vi "CRYGet Weight Array Value.vi"(8 "spectrum type":enum16{"Power", "Amplitude"}(ring), 9 "dB On (T)":bool=TRUE, 10 "frequency [Hz]":dbl=1000.0 min=0.0 format="%.2f", 11 "weighting enum":T1(ring)) -> (3 "relative response level":dbl format="%.2f")   [LabVIEW 2013]
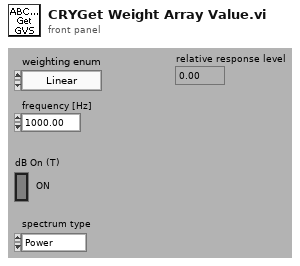
[diagram p1: front panel]
types:
  T1 = enum16{"Linear", "A-weighting", "B-weighting", "C-weighting", "ITU-R 468-4", "Dolby", "CCITT", "C-message", "Wb", "Wc", "Wd", "We", "Wf", "Wh", "Wj", "Wk", "Wm", "Undefined"}
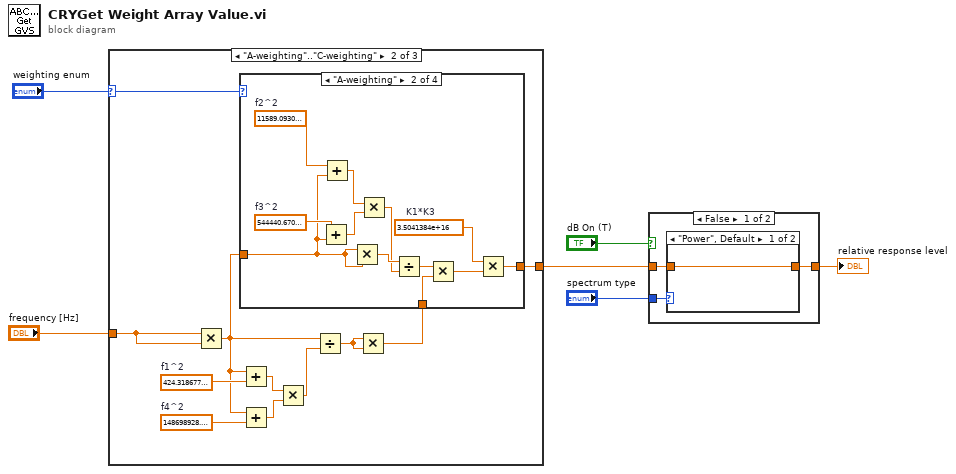
[diagram p0: block diagram]
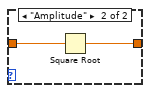
[diagram p2: hidden frame]
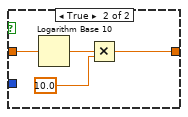
[diagram p3: hidden frame]
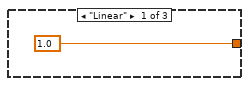
[diagram p4: hidden frame]
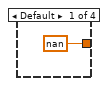
[diagram p5: hidden frame]
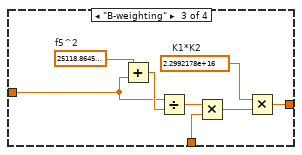
[diagram p6: hidden frame]
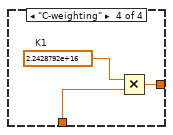
[diagram p7: hidden frame]
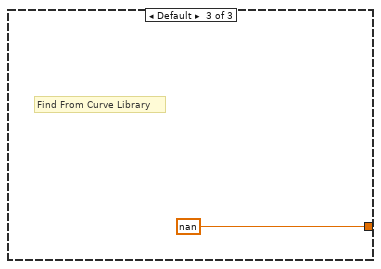
[diagram p8: hidden frame]
diagram:
  n1 = case shown="\"A-weighting\"..\"C-weighting\"" "weighting enum" {
    selector: "weighting enum" -> [_ w9 _]
    tunnel: [1.0 w10 nan] -> w6
    tunnel: "frequency [Hz]" -> [_ w8 _]
    frame "Linear" {
    }
    frame "A-weighting".."C-weighting" {
      w13 = 148698928.24308902  # f4^2
      w14 = 424.31867740600904  # f1^2
      n2 = Multiply(x=w8, y=w8) -> (x*y=w11:dbl)
      n3 = Add(x=w11, y=w14) -> (x+y=w16:dbl)
      n4 = Add(x=w11, y=w13) -> (x+y=w17:dbl)
      n5 = Multiply(x=w16, y=w17) -> (x*y=w15:dbl)
      n6 = Divide(x=w11, y=w15) -> (x/y=w18:dbl)
      n7 = Multiply(x=w18, y=w18) -> (x*y=w12:dbl)
      n8 = case shown="\"A-weighting\"" w9 {
        tunnel: [nan w31 w39 w42] -> w10
        tunnel: w12 -> [_ w29 w36 w41]
        tunnel: w11 -> [_ w20 w34 _]
        frame Default {
        }
        frame "A-weighting" {
          w21 = 544440.6704605728  # f3^2
          w22 = 11589.0930520225  # f2^2
          w25 = 3.5041384e+16  # K1*K3
          n9 = Add(x=w21, y=w20) -> (x+y=w24:dbl)
          n10 = Add(x=w22, y=w20) -> (x+y=w27:dbl)
          n11 = Multiply(x=w20, y=w20) -> (x*y=w26:dbl)
          n12 = Multiply(x=w27, y=w24) -> (x*y=w23:dbl)
          n13 = Divide(x=w26, y=w23) -> (x/y=w30:dbl)
          n14 = Multiply(x=w30, y=w29) -> (x*y=w28:dbl)
          n15 = Multiply(x=w25, y=w28) -> (x*y=w31:dbl)
        }
        frame "B-weighting" {
          w33 = 25118.8645540624  # f5^2
          w32 = 2.2992178e+16  # K1*K2
          n16 = Add(x=w33, y=w34) -> (x+y=w38:dbl)
          n17 = Divide(x=w34, y=w38) -> (x/y=w37:dbl)
          n18 = Multiply(x=w37, y=w36) -> (x*y=w35:dbl)
          n19 = Multiply(x=w32, y=w35) -> (x*y=w39:dbl)
        }
        frame "C-weighting" {
          w40 = 2.2428792e+16  # K1
          n20 = Multiply(x=w40, y=w41) -> (x*y=w42:dbl)
        }
      }
    }
    frame Default {
      # "Find From Curve Library"
    }
  }
  n21 = case shown="False" "dB On (T)" {
    tunnel: w6 -> [w45 w52]
    tunnel: [w46 w51] -> w3
    tunnel: "spectrum type" -> [w44 _]
    frame False {
      n22 = case shown="\"Power\", Default" w44 {
        tunnel: [w47 w49] -> w46
        tunnel: w45 -> [w47 w48]
        frame "Power", Default {
        }
        frame "Amplitude" {
          n23 = Square Root(x=w48) -> (sqrt(x)=w49:dbl)
        }
      }
    }
    frame True {
      n24 = Logarithm Base 10(1:w52) -> (0:w53:dbl)
      n25 = Multiply(x=w53, y=10.0) -> (x*y=w51:dbl)
    }
  }
  "relative response level" <- w3
